vi "ObtainPriorityQueue.vi"(5 "Max Queue Size (-1, unlimited)":i32=-1, 8 "error in":errorcluster, 10 "# of Priority Levels (5)":u32=5) -> (0 "error out":errorcluster, 3 "PriorityMessageQueue out":refnum<class "PriorityMessageQueue.lvclass">)   [LabVIEW 2009, in "LapDog.Messaging.v2.lvlib" / "PriorityMessageQueue.lvclass"]
doc: "<b>This class is deprecated in version 2.1 and will be removed in version 3.0</b>\n\nCreates a Priority Queue object. Priority levels are zero based. If a queue is created with 5 priority levels, the actual priority numbers are 0, 1, 2, 3, and 4. Lower numbered priorties are always returned before higher numbered priorities.\n\nMax Queue Size restricts the number of messages allowed at each priority level. The total number of messages the Priority Queue can hold is equal to the max queue size multiplied by the number of priority levels."
uses:
  PriorityMessageQueue.lvclass
  MessageObject/Message.lvclass
  PriorityMessageQueue.lvclass/PriorityMessageQueue.ctl
panel:
  out "Created New?":bool
  in  "Create If Not Found? (T)":bool=TRUE
  in  "Queue Name":string
  # "The Queue Name, Create If Not Found, and Created New have been disconnected from the front panel while I figure out how to best implement a named priority queue."
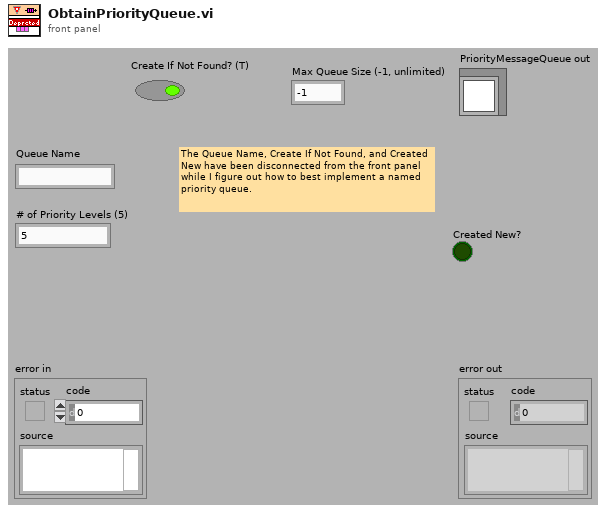
[diagram p1: front panel]
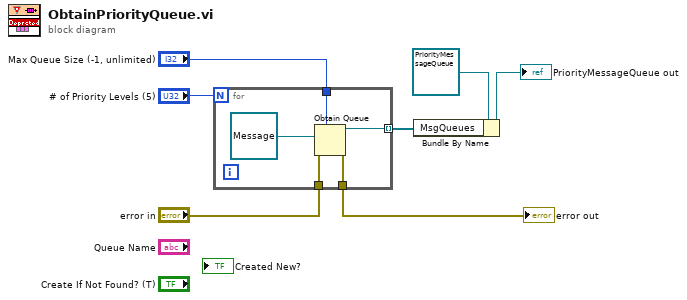
[diagram p0: block diagram]
diagram:
  n1 = for {
    N: "# of Priority Levels (5)" -> [_]
    tunnel: "error in" -> [w12]
    tunnel: [w11] -> w6
    tunnel: [w9] -> w3 mode=indexing
    tunnel: "Max Queue Size (-1, unlimited)" -> [w8]
    n2 = Obtain Queue(max queue size (-1, unlimited)=w8, element data type=refnum<class "Message.lvclass"> refnum ("MessageLibrary.lvlib:Message"), error in (no error)=w12) -> (queue out=w9:refnum<queue>, error out=w11:errorcluster)  [unwired: 2 in, 1 out]
  }
  "error out" <- w6
  n3 = Bundle By Name(cluster=refnum<class "PriorityMessageQueue.lvclass"> refnum ("PriorityMessageQueue in"), "MsgQueues"=w3) -> (→"PriorityMessageQueue out":refnum<class "PriorityMessageQueue.lvclass">)
